vi "oa_Simple Sample Rate Conversion (Continuous) (1 Channel).vi"(0 "even angle signal in":cluster{"r0":dbl, "dr":dbl, "Y":dbl[]}={"r0"=0.0, "dr"=1.0, "Y"=[]} {"r0" format="%.2p"; "dr" format="%.2p"; "Y" format="%.2f"}, 1 "reset? (T)":bool=TRUE, 5 "dr":dbl=1.0 format="%.2p", 7 "interpolation mode":u16(ring)=1 items=["coerce", "linear", "spline", "FIR filter"], 9 "even angle position info":T1, 11 "error in (no error)":errorcluster) -> (4 "even angle signal out":cluster{"r0":dbl, "dr":dbl, "Y":dbl[]}={"r0"=0.0, "dr"=1.0, "Y"=[]} {"r0" format="%.2p"; "dr" format="%.2p"; "Y" format="%.2f"}, 6 "out even angle position info":T1, 15 "error out":errorcluster)   [LabVIEW 2017, in "SoundVib_OAUtility.lvlib"]
uses:
  <vilib>/addons/Sound and Vibration/Order Analysis/Utility/SoundVib_OAUtility.lvlib
  <vilib>/addons/Sound and Vibration/Order Analysis/Misc/OAT Position Info.ctl
  <vilib>/measure/maresamp.llb/Resample Waveform (continuous, t0 DBL).vi
  <vilib>/measure/NI_MAPro.lvlib
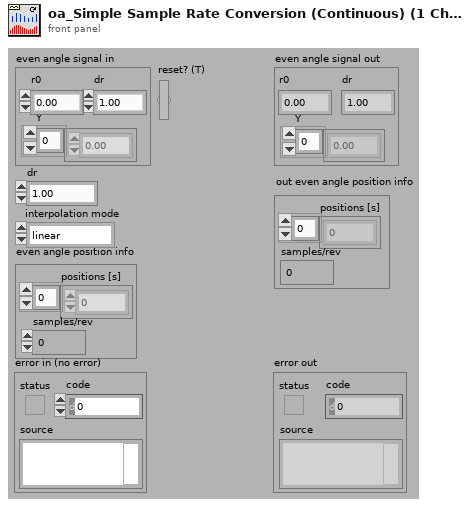
[diagram p1: front panel]
types:
  T1 = typedef "OAT Position Info.ctl" = cluster{"positions [s]":dbl[], "samples/rev":dbl}
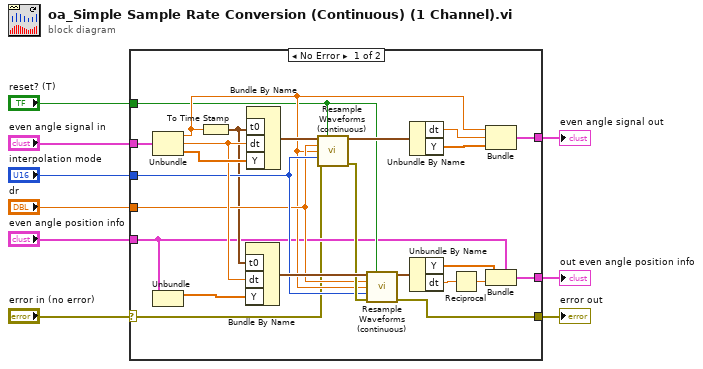
[diagram p0: block diagram]
diagram:
  n1 = case shown="No Error" "error in (no error)" {
    selector: "error in (no error)" -> [w10 w36]
    tunnel: "even angle signal in" -> [w22 w35]
    tunnel: "interpolation mode" -> [w21 _]
    tunnel: "dr" -> [w20 _]
    tunnel: "reset? (T)" -> [w18 _]
    tunnel: [w16 w36] -> w5
    tunnel: [w14 w35] -> w4
    tunnel: [w13 w34] -> w3
    tunnel: "even angle position info" -> [w12 w34]
    frame No Error {
      n2 = Unbundle(w22) -> ("r0"=w19:dbl, "dr"=w23:dbl, "Y"=w24:dbl[])
      n3 = Unbundle(w12) -> ("positions [s]"=w11:dbl[])  [unwired: 1 out]
      n4 = To Time Stamp(1:w19) -> (0:w15:timestamp)
      n5 = Bundle By Name("t0"=w15, "dt"=w23, "Y"=w11) -> (w30:waveform(dbl))  [unwired: 1 in]
      n6 = Bundle By Name("t0"=w15, "dt"=w23, "Y"=w24) -> (w33:waveform(dbl))  [unwired: 1 in]
      n7 = call-poly <vilib>:"Resample Waveforms (continuous).vi"("waveform in"=w33, "reset"=w18, "dt"=w20, "t0"=w19, "interpolation mode"=w21, "error in (no error)"=w10) -> ("resampled waveform out"=w32:waveform(dbl), "error out"=w29:errorcluster)  [unwired: 5 in, 3 out]
      n8 = call-poly <vilib>:"Resample Waveforms (continuous).vi"("waveform in"=w30, "reset"=w18, "dt"=w20, "t0"=w19, "interpolation mode"=w21, "error in (no error)"=w29) -> ("resampled waveform out"=w28:waveform(dbl), "error out"=w16:errorcluster)  [unwired: 5 in, 3 out]
      n9 = Unbundle By Name(w32) -> ("dt"=w31:dbl, "Y"=w25:dbl[])
      n10 = Unbundle By Name(w28) -> ("Y"=w17:dbl[], "dt"=w27:dbl)
      n11 = Reciprocal(x=w27) -> (1/x=w26:dbl)
      n12 = Bundle("r0"=w19, "dt"=w31, "Y"=w25) -> (w14:cluster{"r0":dbl, "dt":dbl, "Y":dbl[]})  [unwired: 1 in]
      n13 = Bundle(cluster=w12, "positions [s]"=w17, "samples/rev"=w26) -> (w13:T1)
    }
    frame Error {
    }
  }
  "error out" <- w5
  "even angle signal out" <- w4
  "out even angle position info" <- w3
